vi "Terminal-Alert-Init.vi"   [LabVIEW 2014]
types:
  T1 = cluster{"报警级别":string, "报警系统":string, "报警详情":string, "备注":string}
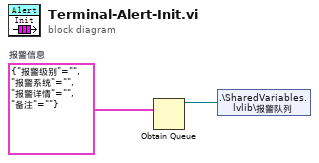
[diagram p0: block diagram]
diagram:
  w2 = T1 {"报警级别"="", "报警系统"="", "报警详情"="", "备注"=""}  # 报警信息
  n1 = Obtain Queue(element data type=w2) -> (queue out=w1:refnum<queue>)  [unwired: 4 in, 2 out]
  n2 = shared-variable ".\\SharedVariables.lvlib\\报警队列"(w1) -> ()  [unwired: 1 in, 1 out]
